vi "Init.vi"(8 "error in (no error)":errorcluster, 10 "Address":string, 11 "Jiaxin_Stepper_Controller in":refnum<class "Jiaxin_Stepper_Controller.lvclass">) -> (0 "error out":errorcluster, 3 "Jiaxin_Stepper_Controller out":refnum<class "Jiaxin_Stepper_Controller.lvclass">)   [LabVIEW 2023, in "Jiaxin_Stepper_Controller.lvlib" / "Jiaxin_Stepper_Controller.lvclass"]
uses:
  Jiaxin_Stepper_Controller.lvclass
  <vilib>/ActorFramework/Actor/Actor.lvclass
  typedefs/instrumentType.ctl
  typedefs/typedefs.lvlib
  typedefs/InstrumentData.ctl
  Jiaxin_Stepper_Controller.lvlib
  Interfaces/InitDeinitInterface/InitDeinitComm Messages/InitDone Msg/InitDone Msg.lvclass
  Plasmionique/MB Master/MB_Master_Serial/MB_Master_Serial.lvclass
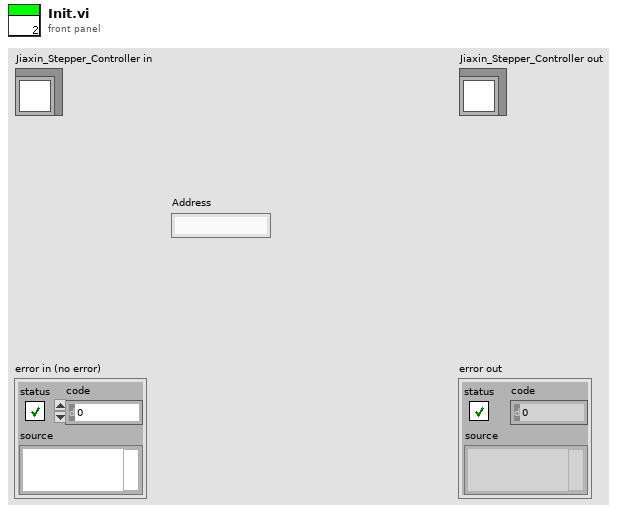
[diagram p1: front panel]
types:
  T1 = typedef "typedefs.lvlib/InstrumentData.ctl" = cluster{"Instr Error":errorcluster, "Address":cluster{"address type":enum16{"VISA", "Index"}, "Address":string, "instrument type":T2}, "CurrentState":cluster{"Initialized":bool, "Connected":bool, "Running":bool, "Error":bool}}
  T2 = typedef "typedefs.lvlib/instrumentType.ctl" = enum16{"Spectrometer", "Camera", "Stepper", "Piezo"}
  T3 = cluster{"baud rate (bps)":u32, "stop bits":u16, "parity":u16, "flow control":u16, "timeout":u32, "retries":i32}
  T4 = cluster{"address type":enum16{"VISA", "Index"}, "Address":string, "instrument type":T2}
  T5 = cluster{"Instr Error":errorcluster, "Address":cluster{"address type":enum16{"VISA", "Index"}, "Address":string, "instrument type":T2}}
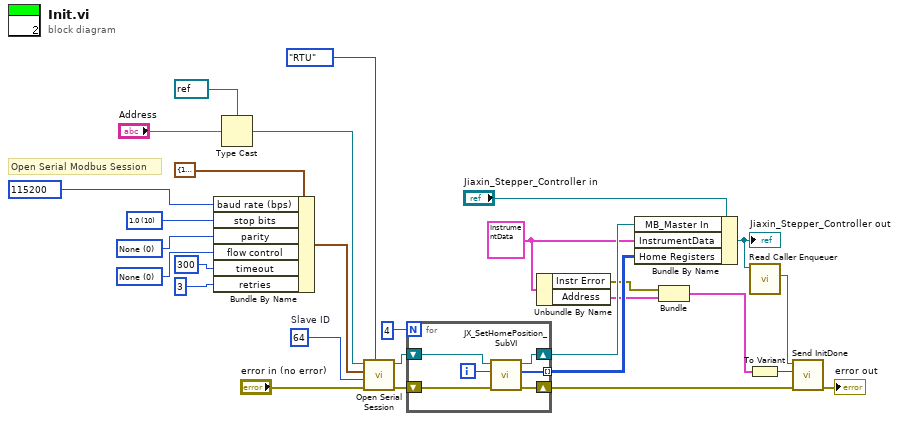
[diagram p0: block diagram]
diagram:
  w5 = T1 {"Instr Error"={"status"=FALSE, "code"=0, "source"=""}, "Address"={"address type"=enum."VISA", "Address"="", "instrument type"=enum."Spectrometer"}, "CurrentState"={"Initialized"=FALSE, "Connected"=FALSE, "Running"=FALSE, "Error"=FALSE}} ("InstrumentData")
  w22 = u32 115200 items=["9600"=9600, "19200"=19200, "38400"=38400, "57600"=57600, "115200"=115200, "460800"=460800, "921600"=921600] ("Baud Rate (bps)")
  w23 = u16 10 items=["1.0"=10, "1.5"=15, "2.0"=20] ("Stop Bits")
  w24 = u16 0 items=["None", "Odd", "Even", "Mark", "Space"] ("Parity")
  w25 = u16 0 items=["None", "XON/XOFF", "RTS/CTS", "XON/XOFF & RTS/CTS", "DTR/DSR", "XON/XOFF & DTR/DSR"] ("Flow Control")
  w28 = u8 64  # Slave ID
  # "Open Serial Modbus Session"
  n1 = Bundle By Name(cluster=T3 {"baud rate (bps)"=19200, "stop bits"=10, "parity"=0, "flow control"=0, "timeout"=1000, "retries"=1} ("Serial Config"), "baud rate (bps)"=w22, "stop bits"=w23, "parity"=w24, "flow control"=w25, "timeout"=u32 300 ("Timeout (ms)"), "retries"=3 ("Retries")) -> (w21:T3)
  n2 = Type Cast(type=refnum<visa-resource-name> refnum ("VISA Resource"), x="Address") -> (*(type *) &x=w15:refnum<visa-resource-name>)
  n3 = call "Open Serial Session.vi"("Mode (RTU)"=enum16{"RTU", "ASCII"}."RTU", "Error in"="error in (no error)", "Slave ID"=w28, "Serial Config"=w21, "VISA Resource"=w15) -> ("Error out"=w10:errorcluster, "MB_Serial session"=w11:refnum<class "MB_Master_Serial.lvclass">)  [unwired: 5 in]
  n4 = for {
    N: 4 -> [_]
    shift-right: [w33] -> w9
    shift-left: w11 -> [w35]
    shift-right: [w32] -> w8
    shift-left: w10 -> [w34]
    tunnel: [w31] -> w6 mode=indexing
    i -> [w30]
    n5 = call "JX_SetHomePosition_SubVI.vi"("error in (no error)"=w34, "channel"=w30, "Jiaxin_Stepper_Controller.lvlib:MB Serial Master:MB_Master"=w35) -> ("error out"=w32:errorcluster, "Registers"=w31:u16[], "Jiaxin_Stepper_Controller.lvlib:MB Serial Master:MB_Master"=w33:refnum<class "MB_Master_Serial.lvclass">)  [unwired: 6 in]
  }
  n6 = Unbundle By Name(w5) -> ("Instr Error"=w4:errorcluster, "Address"=w3:T4)
  n7 = Bundle By Name(cluster="Jiaxin_Stepper_Controller in", "MB_Master In"=w9, "InstrumentData"=w5, "Home Registers"=w6) -> (w14:refnum<class "Jiaxin_Stepper_Controller.lvclass">)
  "Jiaxin_Stepper_Controller out" <- w14
  n8 = Bundle("Instr Error"=w4, "Address"=w3) -> (w2:T5)  [unwired: 1 in]
  n9 = call <vilib>:"Read Caller Enqueuer.vi"("Actor"=w14) -> ("Caller Enqueuer"=w13:refnum<class "Message Enqueuer.lvclass">)  [unwired: 10 in]
  n10 = To Variant(anything=w2) -> (Variant=w1:variant)
  n11 = call "Send InitDone.vi"("error in (no error)"=w8, "Variant"=w1, "Message Enqueuer"=w13) -> ("error out"=→"error out":errorcluster)  [unwired: 7 in, 1 out]
